vi "Key Press Sequence.vi"(8 "error in (no error)":errorcluster, 11 "Vk":u16) -> (0 "error out":errorcluster, 3 "Key Press Array":u8[][](array[numeric]))   [LabVIEW 2020, in "MacroAssert.lvlib" / "Win Util.lvlib"]
uses:
  Win Util.lvlib
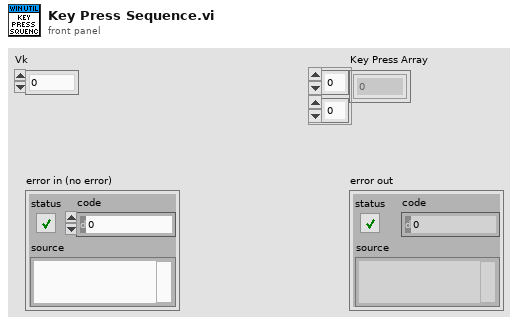
[diagram p1: front panel]
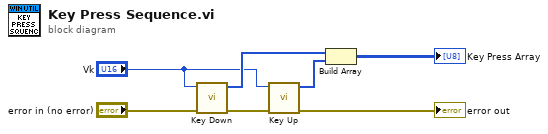
[diagram p0: block diagram]
diagram:
  n1 = call "Key Down.vi"("error in (no error)"="error in (no error)", "Vk"="Vk") -> ("error out"=w2:errorcluster, "Input"=w6:u8[])  [unwired: 8 in]
  n2 = call "Key Up.vi"("error in (no error)"=w2, "Vk"="Vk") -> ("error out"=→"error out":errorcluster, "Input"=w5:u8[])  [unwired: 8 in]
  n3 = Build Array(w6, w5) -> (→"Key Press Array":u8[][])
